vi "simulation.vi"(1 "Stop signaller":refnum<class "Signaller.lvclass">, 2 "Simulation config action queue":refnum<queue>, 3 "Frequency refnum":refnum<vi>, 4 "Data input file refnum":refnum<vi>) -> ()   [LabVIEW 2019]
uses:
  Fit Parameters.ctl
  Physical Constants.ctl
  Internal Parameters.ctl
  System parameters.ctl
  Motor controller/Signaller/Signaller.lvclass
  <vilib>/Platform/TimedLoop/XDataNode/timing_clust.ctl
  <vilib>/Platform/TimedLoop/XDataNode/nitl_modes.ctl
  <vilib>/Platform/TimedLoop/XDataNode/wakeup.ctl
  <vilib>/Platform/TimedLoop/scheduler/LVUserAPI/_suppVIs/Create_1kHz_TSource.vi
  <vilib>/Utility/file.llb/Write Delimited Spreadsheet (string).vi
  <vilib>/Utility/config.llb/Read Key (Path).vi
  <vilib>/Utility/config.llb/Read Key (Boolean).vi
  <vilib>/Utility/config.llb/Read Key (Double).vi
  <vilib>/Utility/config.llb/Read Key (U32).vi
  <vilib>/Utility/config.llb/Read Key (I32).vi
  <vilib>/Utility/config.llb/Write Key (Path).vi
  <vilib>/Utility/config.llb/Write Key (Boolean).vi
  <vilib>/Utility/config.llb/Write Key (Double).vi
  <vilib>/Utility/config.llb/Write Key (U32).vi
  <vilib>/Utility/config.llb/Write Key (I32).vi
  <vilib>/platform/TimedLoop/XDataNode/XDataNode.xnode
  <vilib>/Platform/TimedLoop/XDataNode/XDNodeRunTimeDep.lvlib
  <vilib>/Utility/config.llb/NI_LVConfig.lvlib
panel:
  in  "Precision":i32=100 min=1
  in  "Sweep error":dbl=0.01 min=0.0 format="%#_13g"
  out "Start time":timestamp
  out "Polarization (unfuzzed)":dbl
  in  "Thermal fluctuations":dbl=0.01 min=0.0
  out "Pn (noisy)":dbl
  in  "System parameters":T1={"Frequency (GHz)"=140.2, "System temperature (K)"=1.0, "Beam current (nA)"=100.0}
  out "Internal parameters":T2={"Pe"=-1.0, "Pn"=0.0, "Alpha"=0.0, "Beta"=0.0, "C"=0.000136073, "Phi"=0.0, "Pe0"=-1.0, "Dose"=0.0, "Temperature"=1.0}
  in  "Physical constants":T3={"T1e (s)"=0.03, "T1n (s)"=1500.0}
  in  "Fit parameters":T4={"A"=0.572086, "S"=0.0835606, "M1"=140.286, "M2"=140.486}
  in  "Launch fit parameters chooser":bool
  out "Elapsed time (s)":dbl
  in  "Reset simulation":bool
  in  "Paused":bool=TRUE
  out "Current time (simulated)":timestamp format="%<%H:%M:%S\n%B %d, %Y>T"
  in  "Stop simulation":bool
  in  "Data output file":path
  out "Polarization":dbl
  in  "Beam on":bool
  in  "Time per second (s)":dbl=1.0
  out "Seconds until next data":u32
  in  "# Sweeps":u32=250
  in  "Add 30 minutes":bool
  in  "30 minutes":bool
  in  "15 minutes":bool
  in  "5 minutes":bool
  in  "Time scale (min)":i64=5 min=1
  out "Polarization vs time":cluster{timestamp[], dbl[]}(graph)
  # "Advanced data and controls"
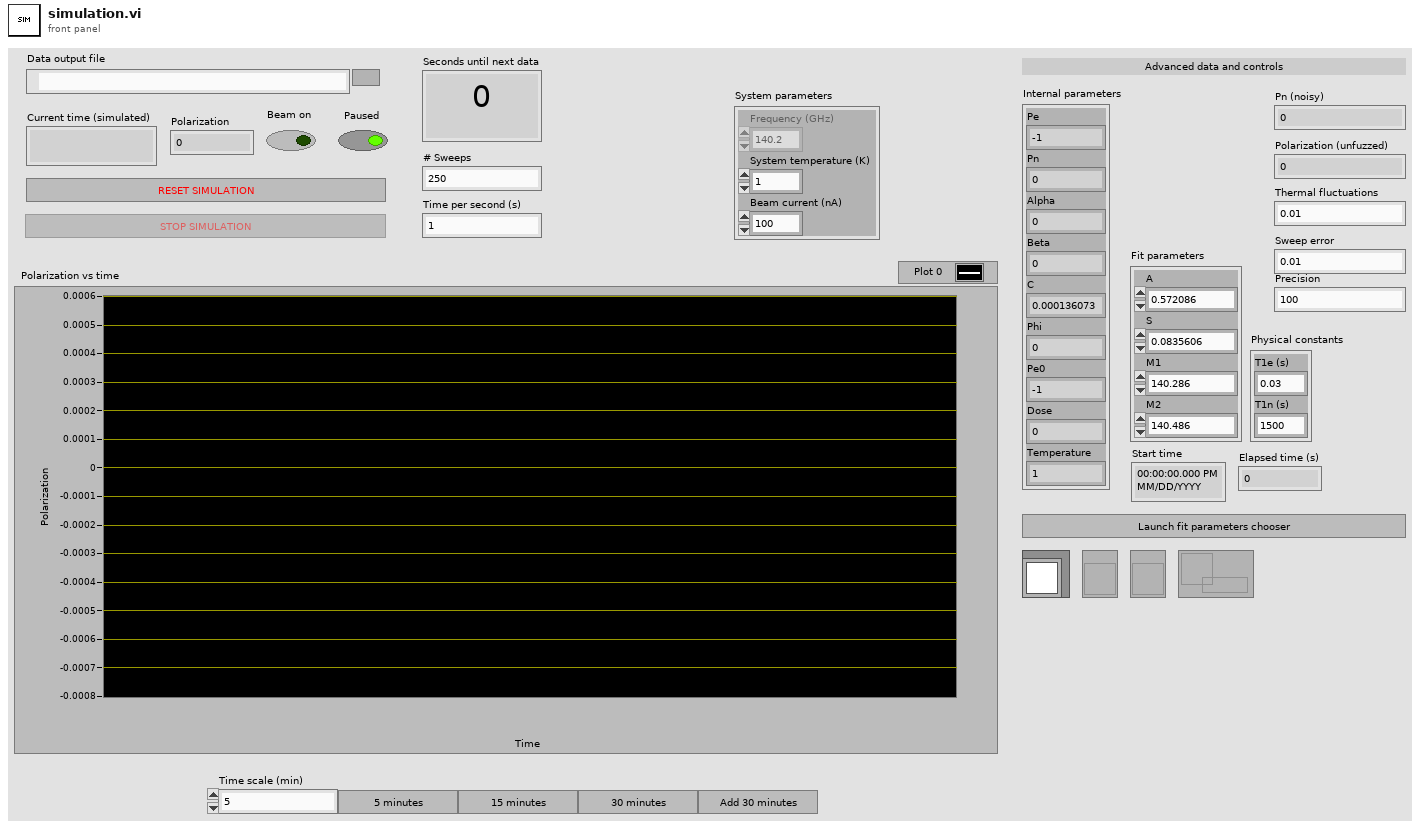
[diagram p1: front panel]
types:
  T1 = typedef "System parameters.ctl" = cluster{"Frequency (GHz)":dbl, "System temperature (K)":dbl, "Beam current (nA)":dbl}
  T2 = typedef "Internal Parameters.ctl" = cluster{"Pe":dbl, "Pn":dbl, "Alpha":dbl, "Beta":dbl, "C":dbl, "Phi":dbl, "Pe0":dbl, "Dose":dbl, "Temperature":dbl}
  T3 = typedef "Physical Constants.ctl" = cluster{"T1e (s)":dbl, "T1n (s)":dbl}
  T4 = typedef "Fit Parameters.ctl" = cluster{"A":dbl, "S":dbl, "M1":dbl, "M2":dbl}
  T5 = enum8{"Enabled", "Disabled", "Disabled and Grayed Out"}
  T6 = typedef "Semaphore RefNum" = refnum<k1>
  T7 = typedef "XDNodeRunTimeDep.lvlib/timing_clust.ctl" = cluster{"Expected End [f-1]":u64, "Actual End [f-1]":u64, "Finished Late? [f-1]":bool, "Expected End [i-1]":u64, "Actual End [i-1]":u64, "Finished Late? [i-1]":bool, "Expected Start [i]":u64, "Actual Start [i]":u64, "Expected Start [f]":u64, "Actual Start [f]":u64, "Source Name":string, "Structure Name":string, "Period":i64, "Deadline":i64, "Offset":i64, "Start":i64, "Priority":i32, "Timeout":i32, "Mode":T8, "Wakeup Reason":T9, "Error":errorcluster, "Source Type":string, "Secondary Source Type":string, "Global End Time":u64, "Global Start Time":u64, "Frame Duration":u64, "Iteration Duration":u64, "Assigned CPU":i32, "I/O Scan Engine Mode":u32}
  T8 = typedef "XDNodeRunTimeDep.lvlib/nitl_modes.ctl" = enum32{"No Change", "Process missed periods, maintain original phase", "Discard missed periods, maintain original phase", "Process missed periods, ignore original phase", "Discard missed periods, ignore original phase"}
  T9 = typedef "XDNodeRunTimeDep.lvlib/wakeup.ctl" = enum32{"Normal", "Aborted", "Asynchronous wakeup", "Timing source error", "Timed loop error", "Timeout"}
  T10 = typedef "LVRangeTypeDef.ctl" = cluster{"Minimum":dbl, "Maximum":dbl, "Increment":dbl, "Minor Increment":dbl, "Start":dbl}
  T11 = typedef "NI_LVConfig.lvlib/Config Data RefNum.ctl" = refnum<k1>
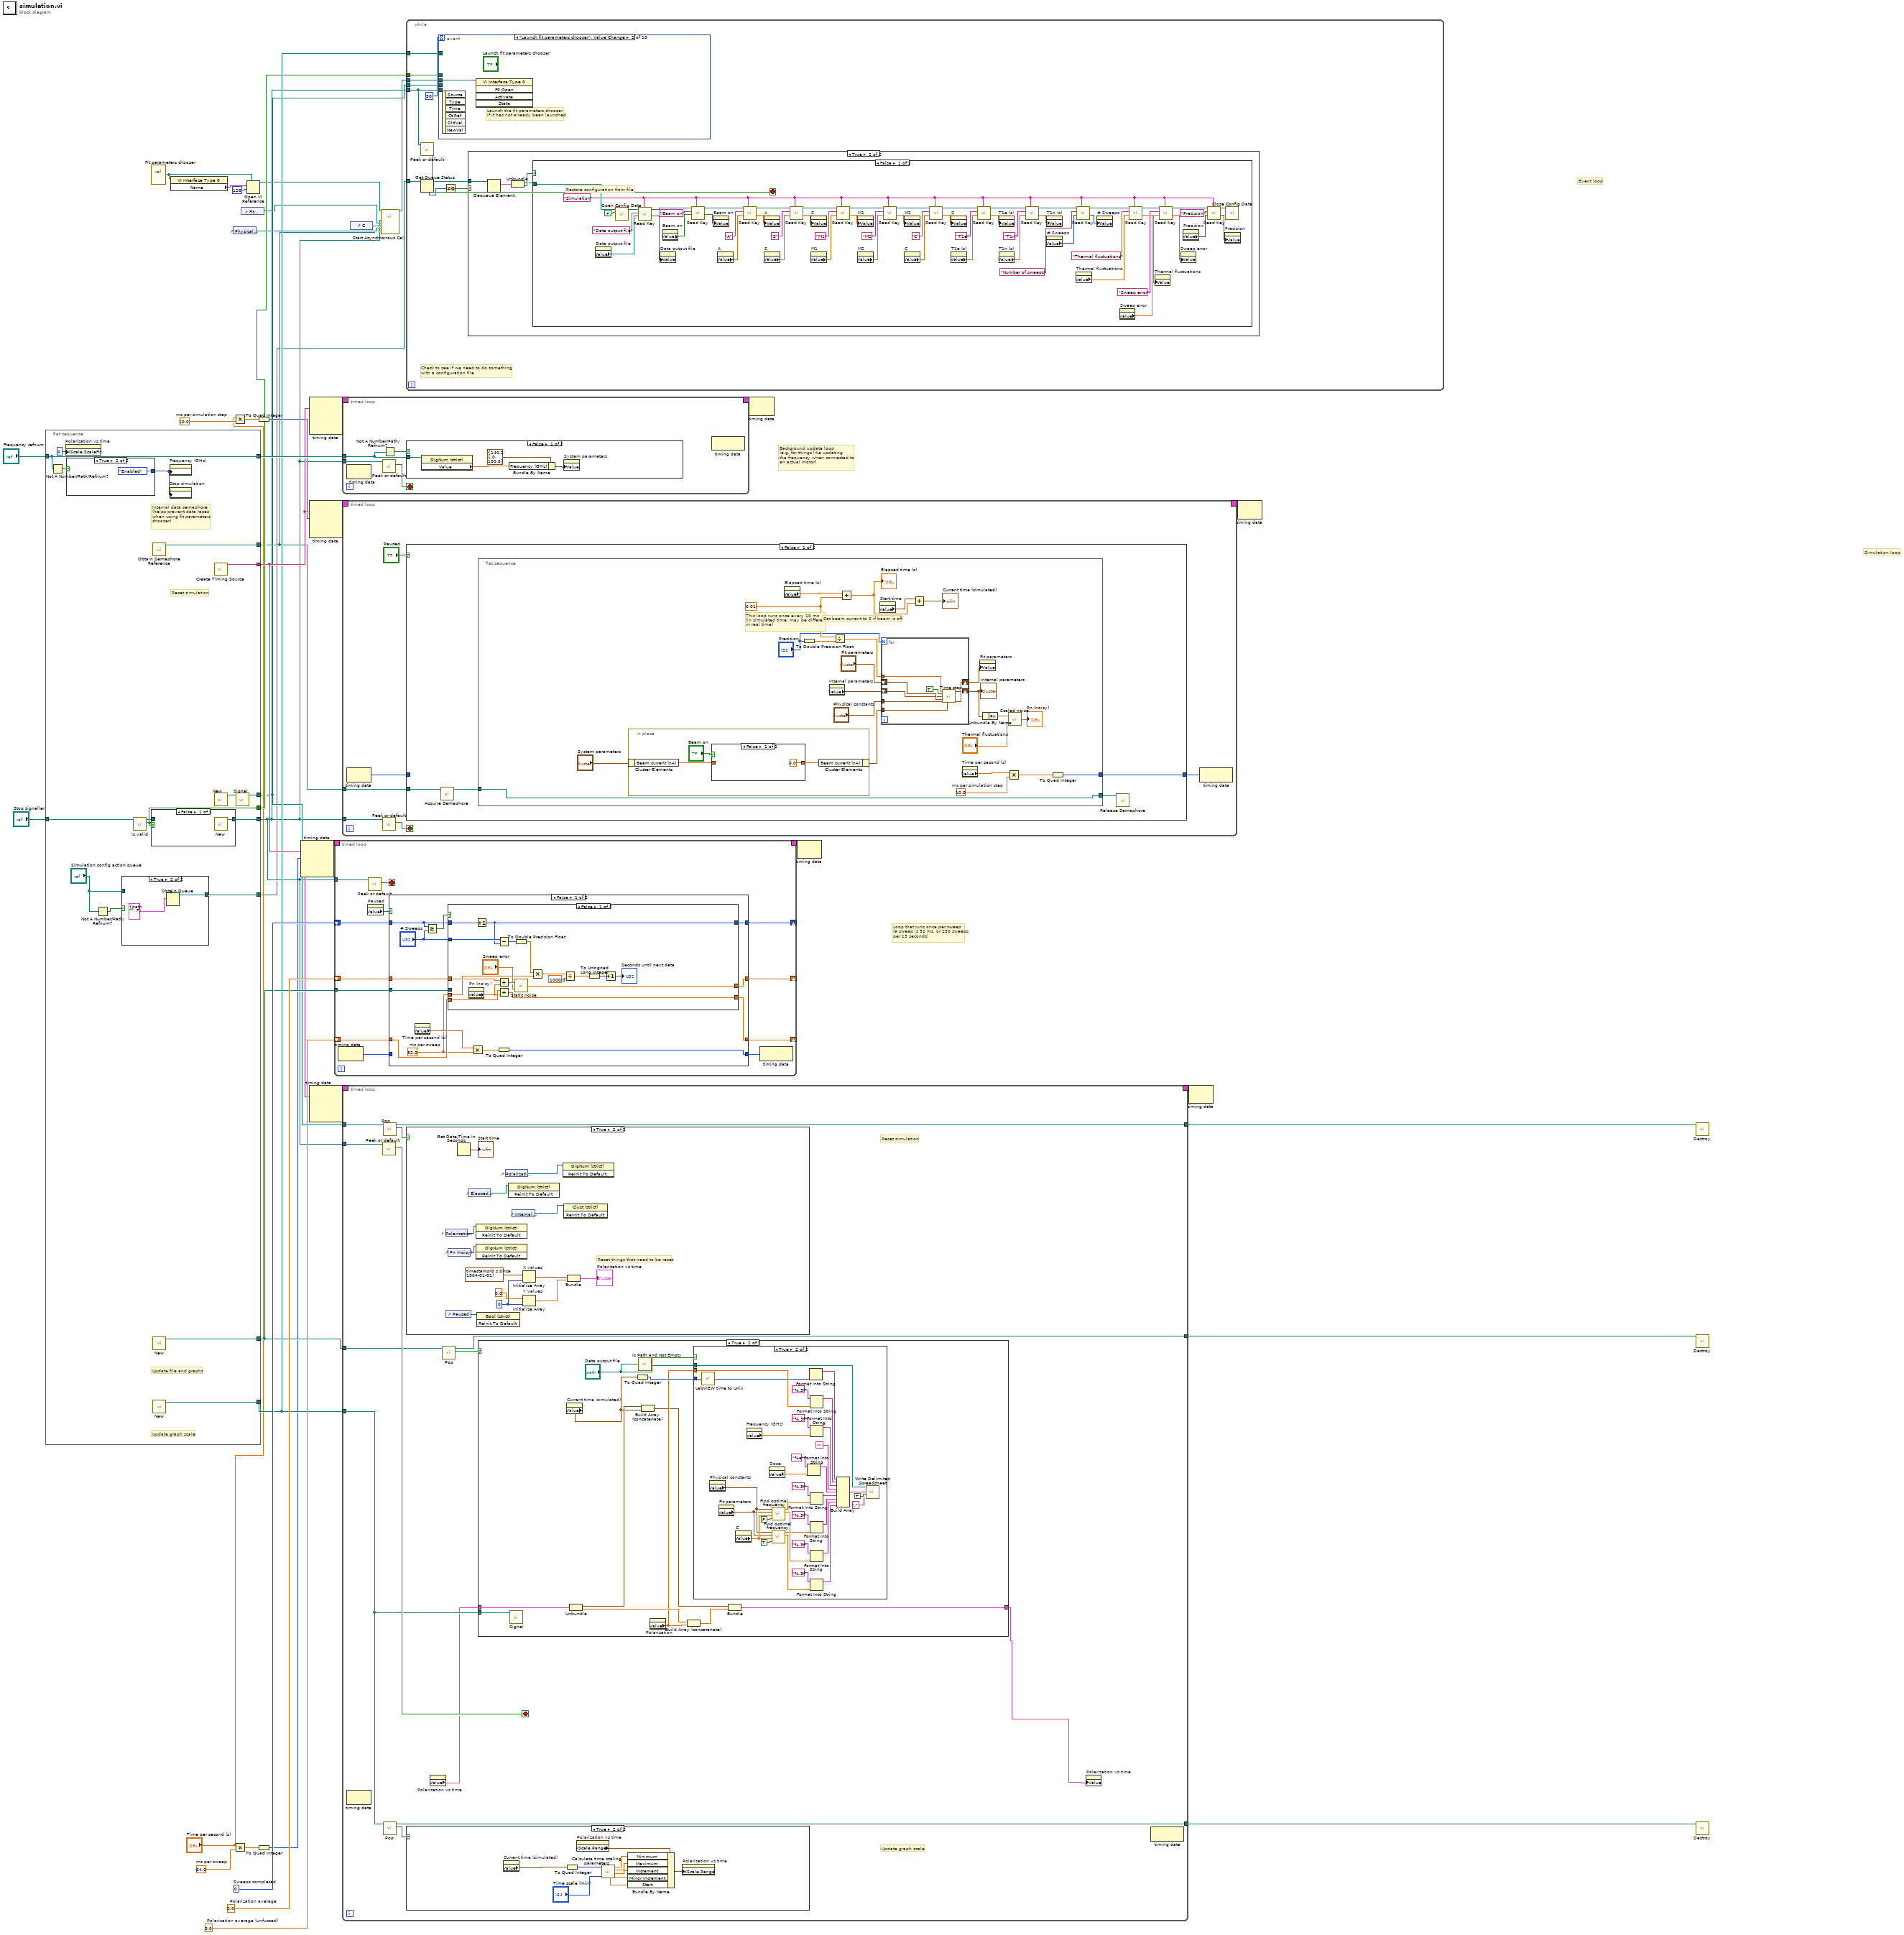
[diagram p0: block diagram]
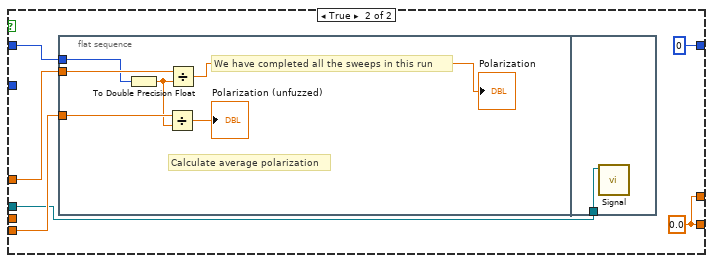
[diagram p6: hidden frame]
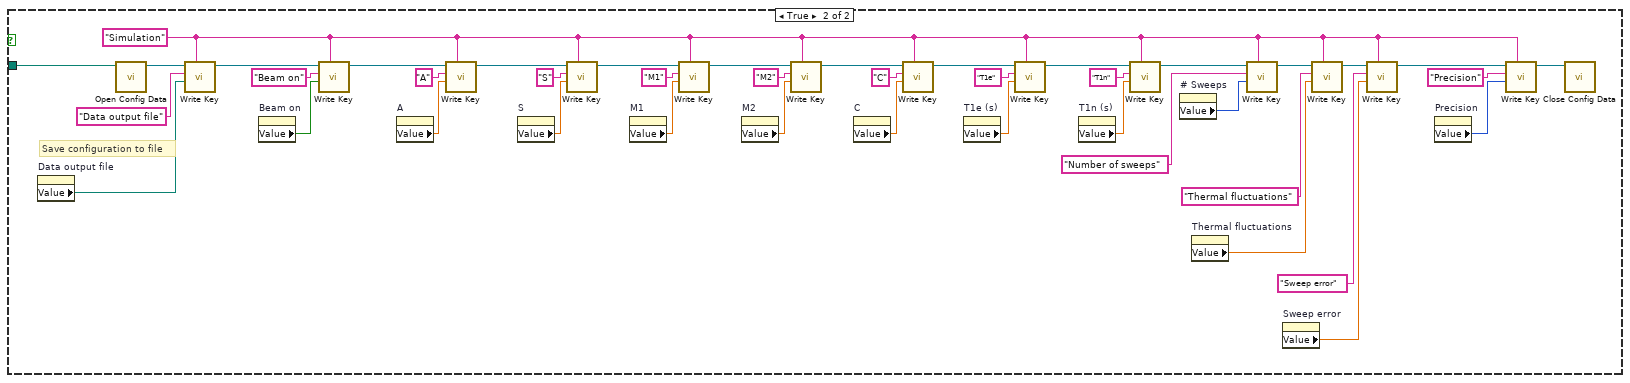
[diagram p12: hidden frame]
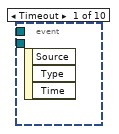
[diagram p13: hidden frame]
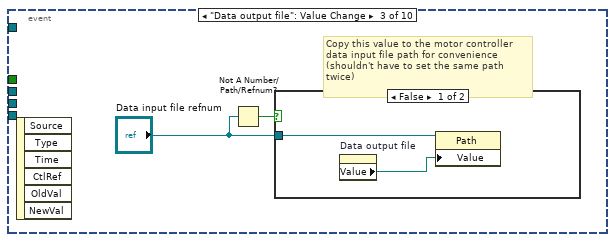
[diagram p14: hidden frame]
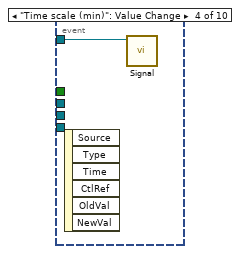
[diagram p16: hidden frame]
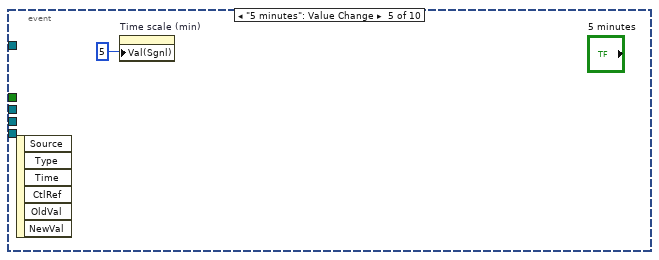
[diagram p17: hidden frame]
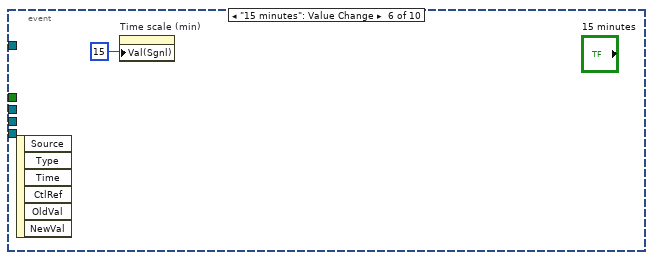
[diagram p18: hidden frame]
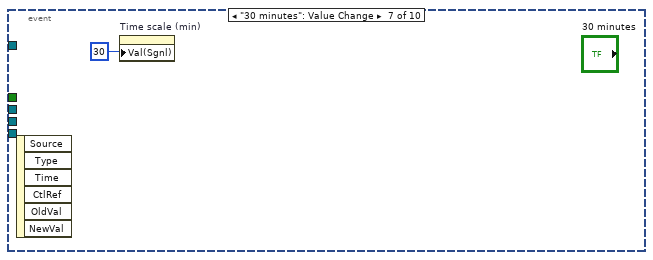
[diagram p19: hidden frame]
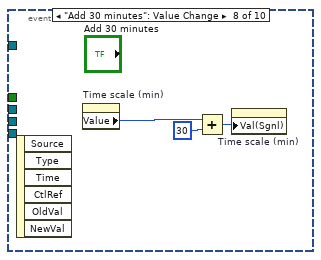
[diagram p20: hidden frame]
diagram:
  w16 = 64.0  # ms per sweep
  w20 = 10.0  # ms per simulation step
  w30 = 0.0  # Polarization average (unfuzzed)
  w31 = 0.0  # Polarization average
  w32 = u32 0  # Sweeps completed
  # "Loop that runs once per sweep\n(a sweep is 52 ms, or 250 sweeps\nper 13 seconds)"
  # "Background update loop\n(e.g. for things like updating\nthe frequency when connected to\nan actual motor)"
  # "Event loop"
  # "Simulation loop"
  n1 = flat-sequence {
    tunnel: "Frequency refnum" -> [w56]
    tunnel: [w48] -> w3
    tunnel: [w56] -> w39
    tunnel: [w53] -> w28
    tunnel: [w52] -> w22
    tunnel: "Stop signaller" -> [w50]
    tunnel: [w51] -> w23
    tunnel: [w47] -> w21
    tunnel: [w45] -> w12
    tunnel: [w44] -> w4
    tunnel: [w42] -> w1
    frame #0 {
      # "Internal data semaphore\n(helps prevent data races\nwhen using fit parameters\nchooser)"
      # "Reset simulation"
      # "Update graph scale"
      # "Update file and graphs"
      n2 = Not A Number/Path/Refnum?(number/path/refnum=w56) -> (NaN/Path/Refnum?=w57:bool)
      n3 = property on="Polarization vs time" class="XYGraph (strict)"("XScale.ScaleFit"=u8 0 ("X Scale.Scale Fit")) -> ()  [unwired: 2 in, 2 out]
      n4 = case shown="True" w57 {
        tunnel: [T5."Disabled and Grayed Out" ("Disabled") T5."Enabled" ("Disabled")] -> w54
        frame False {
        }
        frame True {
        }
      }
      n5 = Not A Number/Path/Refnum?(number/path/refnum="Simulation config action queue") -> (NaN/Path/Refnum?=w43:bool)
      n6 = case shown="True" w43 {
        tunnel: [w58 w59] -> w42
        tunnel: "Simulation config action queue" -> [w58 _]
        frame False {
        }
        frame True {
          n7 = Obtain Queue(element data type=cluster{path, bool} {path "", FALSE}) -> (queue out=w59:refnum<queue>)  [unwired: 4 in, 2 out]
        }
      }
      n8 = call "Is valid.vi"("Signaller in"=w50) -> ("Is valid?"=w47:bool, "Signaller out"=w49:refnum<class "Signaller.lvclass">)  [unwired: 8 in, 1 out]
      n9 = case shown="False" w47 {
        tunnel: w49 -> [_ w62]
        tunnel: [w61 w62] -> w48
        frame False {
          n10 = call "New.vi"() -> ("Signaller out"=w61:refnum<class "Signaller.lvclass">)  [unwired: 11 in]
        }
        frame True {
        }
      }
      n11 = call <vilib>:"Obtain Semaphore Reference.vi"() -> ("semaphore"=w44:T6)  [unwired: 5 in, 2 out]
      n12 = call "New.vi"() -> ("Signaller out"=w53:refnum<class "Signaller.lvclass">)  [unwired: 11 in]
      n13 = call "New.vi"() -> ("Signaller out"=w52:refnum<class "Signaller.lvclass">)  [unwired: 11 in]
      n14 = property on="Frequency (GHz)" class="DigNum (strict)"("DisabledEnum"=w54) -> ()  [unwired: 2 in, 2 out]
      n15 = property on="Stop simulation" class="Bool"("DisabledEnum"=w54) -> ()  [unwired: 2 in, 2 out]
      n16 = call-poly <vilib>:"Create Timing Source.vi"() -> ("name (out)"=w51:string)  [unwired: 10 in, 1 out]
      n17 = call "New.vi"() -> ("Signaller out"=w46:refnum<class "Signaller.lvclass">)  [unwired: 11 in]
      n18 = call "Signal.vi"("Signaller in"=w46) -> ("Signaller out"=w45:refnum<class "Signaller.lvclass">)  [unwired: 9 in, 1 out]
    }
  }
  n19 = vi-ref "Fit parameters chooser.vi"() -> (w7:refnum<vi>)
  n20 = property class="VI Interface Type 0"(reference=w7) -> ("Name"=w8:string)  [unwired: 1 in, 2 out]
  n21 = control-ref of="Physical constants"() -> (w11:refnum<vi>)
  n22 = Multiply(x="Time per second (s)", y=w20) -> (x*y=w19:dbl)
  n23 = Multiply(x="Time per second (s)", y=w16) -> (x*y=w15:dbl)
  n24 = control-ref of="Fit parameters"() -> (w9:refnum<vi>)
  n25 = Open VI Reference(type specifier VI Refnum (for type only)=w7, vi path=w8, options=128) -> (vi reference=w5:refnum<vi>)  [unwired: 3 in, 1 out]
  n26 = To Quad Integer(1:w19) -> (0:w18:i64)
  n27 = To Quad Integer(1:w15) -> (0:w14:i64)
  n28 = node-c288(w23, w14) -> (w34:T7)  [unwired: 2 in]
  n29 = node-c288(w23) -> (w36:T7)  [unwired: 3 in]
  n30 = node-c288(w23, w18) -> (w38:T7)  [unwired: 2 in]
  n31 = node-c288(w23) -> (w27:T7)  [unwired: 3 in]
  n32 = timed-loop {
    timing: w34 -> [_]
    timing-out: [_] -> w33
    tunnel: w3 -> [w75]
    shift-right: [w73] -> _
    shift-left: w32 -> [w74]
    shift-right: [w71] -> _
    shift-left: w31 -> [w72]
    shift-right: [w69] -> _
    shift-left: w30 -> [w70]
    tunnel: w28 -> [w68]
    stop <- w76 stop-if-true
    n33 = node-c288() -> (w65:i64)  [unwired: 1 in]
    n34 = property on="Paused" class="Bool (strict)"() -> ("Value"=w66:bool)  [unwired: 2 in, 2 out]
    n35 = call "Peek or default.vi"("Signaller in"=w75) -> ("Has signal?"=w76:bool)  [unwired: 8 in, 2 out]
    n36 = case shown="False" w66 {
      tunnel: w74 -> [w88 w124]
      tunnel: [w87 w124] -> w73
      tunnel: w72 -> [w85 w123]
      tunnel: [w84 w123] -> w71
      tunnel: w70 -> [w83 w122]
      tunnel: [w82 w122] -> w69
      tunnel: w68 -> [w81 _]
      tunnel: [w79 w121] -> w67
      tunnel: w65 -> [_ w121]
      frame False {
        w77 = 52.0  # ms per sweep
        n37 = property on="Time per second (s)" class="DigNum (strict)"() -> ("Value"=w80:dbl)  [unwired: 2 in, 2 out]
        n38 = Greater Or Equal?(x=w88, y="# Sweeps") -> (x >= y?=w89:bool)
        n39 = case shown="False" w89 {
          tunnel: w88 -> [w106 w111]
          tunnel: [w105 u32 0] -> w87
          tunnel: "# Sweeps" -> [w107 _]
          tunnel: w85 -> [w103 w112]
          tunnel: [w101 w109] -> w84
          tunnel: w83 -> [w99 w110]
          tunnel: [w97 w109] -> w82
          tunnel: w81 -> [_ w108]
          tunnel: w77 -> [w95 _]
          frame False {
            n40 = property on="Pn (noisy)" class="DigNum (strict)"() -> ("Value"=w98:dbl)  [unwired: 2 in, 2 out]
            n41 = Increment(x=w106) -> (x+1=w105:u32)
            n42 = Subtract(x=w107, y=w105) -> (x-y=w96:u32)
            n43 = Add(x=w103, y=w98) -> (x+y=w102:dbl)
            n44 = Add(x=w99, y=w98) -> (x+y=w97:dbl)
            n45 = To Double Precision Float(number=w96) -> (double precision float=w94:dbl)
            n46 = call "Static noise.vi"("Fraction"="Sweep error", "Input"=w102) -> ("Output with noise"=w101:dbl)
            n47 = Multiply(x=w94, y=w95) -> (x*y=w93:dbl)
            n48 = Divide(x=w93, y=1000.0) -> (x/y=w91:dbl)
            n49 = To Unsigned Long Integer(number=w91) -> (unsigned 32bit integer=w90:u32)
            n50 = Increment(x=w90) -> (x+1=→"Seconds until next data":u32)
          }
          frame True {
            w109 = 0.0
            n51 = flat-sequence {
              tunnel: w112 -> [w119]
              tunnel: w111 -> [w118]
              tunnel: w110 -> [w116]
              tunnel: w108 -> [w120]
              frame #0 {
                # "Calculate average polarization"
                # "We have completed all the sweeps in this run"
                n52 = To Double Precision Float(number=w118) -> (double precision float=w115:dbl)
                n53 = Divide(x=w116, y=w115) -> (x/y=→"Polarization (unfuzzed)":dbl)
                n54 = Divide(x=w119, y=w115) -> (x/y=→"Polarization":dbl)
              }
              frame #1 {
                n55 = call "Signal.vi"("Signaller in"=w120) -> ()  [unwired: 9 in, 2 out]
              }
            }
          }
        }
        n56 = Multiply(x=w80, y=w77) -> (x*y=w78:dbl)
        n57 = To Quad Integer(1:w78) -> (0:w79:i64)
      }
      frame True {
      }
    }
    n58 = node-c288(w67) -> ()  [unwired: 1 out]
  }
  n59 = timed-loop {
    tunnel: w39 -> [w132]
    tunnel: w3 -> [w130]
    timing: w36 -> [_]
    timing-out: [_] -> w35
    stop <- w131 stop-if-true
    n60 = node-c288() -> ()  [unwired: 1 in, 1 out]
    n61 = call "Peek or default.vi"("Signaller in"=w130) -> ("Has signal?"=w131:bool)  [unwired: 8 in, 2 out]
    n62 = Not A Number/Path/Refnum?(number/path/refnum=w132) -> (NaN/Path/Refnum?=w133:bool)
    n63 = case shown="False" w133 {
      tunnel: w132 -> [w139 _]
      frame False {
        n64 = property class="DigNum (strict)"(reference=w139) -> ("Value"=w136:dbl)  [unwired: 1 in, 2 out]
        n65 = Bundle By Name(cluster=T1 {"Frequency (GHz)"=140.2, "System temperature (K)"=1.0, "Beam current (nA)"=100.0} ("System parameters"), "Frequency (GHz)"=w136) -> (w138:T1)
        n66 = property on="System parameters" class="Clust (strict)"("Value"=w138) -> ()  [unwired: 2 in, 2 out]
      }
      frame True {
      }
    }
    n67 = node-c288() -> ()  [unwired: 1 in, 1 out]
  }
  n68 = timed-loop {
    tunnel: w3 -> [w144]
    timing: w38 -> [_]
    timing-out: [_] -> w37
    tunnel: w4 -> [w140]
    stop <- w145 stop-if-true
    n69 = node-c288() -> (w141:i64)  [unwired: 1 in]
    n70 = call "Peek or default.vi"("Signaller in"=w144) -> ("Has signal?"=w145:bool)  [unwired: 8 in, 2 out]
    n71 = case shown="False" "Paused" {
      tunnel: [w149 w186] -> w143
      tunnel: w141 -> [_ w186]
      tunnel: w140 -> [w148 _]
      frame False {
        n72 = call <vilib>:"Acquire Semaphore.vi"("semaphore"=w148) -> ("semaphore out"=w147:T6)  [unwired: 4 in, 2 out]
        n73 = flat-sequence {
          tunnel: [w158] -> w149
          tunnel: w147 -> [w156]
          tunnel: [w156] -> w146
          frame #0 {
            w160 = 10.0  # ms per simulation step
            w153 = 0.01
            # "This loop runs once every 10 ms\n(in simulated time; may be different\nin real time)"
            # "Set beam current to 0 if beam is off"
            n74 = in-place {
              n75 = in-place-cluster #1("System parameters") -> ("Beam current (nA)"=w182:dbl)
              n76 = case shown="False" "Beam on" {
                tunnel: w182 -> [_ w185]
                tunnel: [0.0 ("Beam current (nA)") w185] -> w181
                frame False {
                }
                frame True {
                }
              }
              n77 = in-place-cluster #1("Beam current (nA)"=w181) -> (w165:T1)
            }
            n78 = property on="Elapsed time (s)" class="DigNum (strict)"() -> ("Value"=w172:dbl)  [unwired: 2 in, 2 out]
            n79 = To Double Precision Float(number="Precision") -> (double precision float=w152:dbl)
            n80 = property on="Internal parameters" class="Clust (strict)"() -> ("Value"=w154:T2)  [unwired: 2 in, 2 out]
            n81 = Divide(x=w153, y=w152) -> (x/y=w150:dbl)
            n82 = Add(x=w172, y=w153) -> (x+y=w162:dbl)
            "Elapsed time (s)" <- w162
            n83 = property on="Start time" class="AbsTime (strict)"() -> ("Value"=w163:timestamp)  [unwired: 2 in, 2 out]
            n84 = for {
              N: "Precision" -> [_]
              tunnel: "Physical constants" -> [w180]
              tunnel: w165 -> [w178]
              tunnel: w150 -> [w176]
              shift-right: [w175] -> w157
              shift-left: "Fit parameters" -> [w179]
              shift-right: [w174] -> w155
              shift-left: w154 -> [w173]
              n85 = call "Time step.vi"("Time (s)"=w176, "Microwave on"=TRUE, "Internal parameters in"=w173, "Fit parameters"=w179, "Physical constants"=w180, "System parameters"=w178) -> ("Internal parameters out"=w174:T2, "Fit parameters out"=w175:T4)  [unwired: 8 in]
            }
            "Internal parameters" <- w155
            n86 = Add(x=w163, y=w162) -> (x+y=→"Current time (simulated)":timestamp)
            n87 = property on="Time per second (s)" class="DigNum (strict)"() -> ("Value"=w159:dbl)  [unwired: 2 in, 2 out]
            n88 = property on="Fit parameters" class="Clust (strict)"("Value"=w157) -> ()  [unwired: 2 in, 2 out]
            n89 = Unbundle By Name(w155) -> ("Pn"=w170:dbl)
            n90 = Multiply(x=w159, y=w160) -> (x*y=w161:dbl)
            n91 = call "Scaled noise.vi"("Fraction"="Thermal fluctuations", "Input"=w170) -> ("Output with noise"=→"Pn (noisy)":dbl)
            n92 = To Quad Integer(1:w161) -> (0:w158:i64)
          }
        }
        n93 = call <vilib>:"Release Semaphore.vi"("semaphore"=w146) -> ()  [unwired: 5 in, 2 out]
      }
      frame True {
      }
    }
    n94 = node-c288(w143) -> ()  [unwired: 1 out]
  }
  n95 = timed-loop {
    tunnel: w3 -> [w202]
    tunnel: w28 -> [w201]
    tunnel: [w200] -> w29
    timing: w27 -> [_]
    timing-out: [_] -> w26
    tunnel: w22 -> [w197]
    tunnel: [w198] -> w25
    tunnel: w12 -> [w196]
    tunnel: [w194] -> w13
    stop <- w203 stop-if-true
    # "Update graph scale"
    # "Reset simulation"
    n96 = node-c288() -> ()  [unwired: 1 in, 1 out]
    n97 = call "Peek or default.vi"("Signaller in"=w202) -> ("Has signal?"=w203:bool)  [unwired: 8 in, 2 out]
    n98 = call "Pop.vi"("Signaller in"=w196) -> ("Has signal"=w195:bool, "Signaller out"=w194:refnum<class "Signaller.lvclass">)  [unwired: 8 in, 1 out]
    n99 = call "Pop.vi"("Signaller in"=w197) -> ("Has signal"=w199:bool, "Signaller out"=w198:refnum<class "Signaller.lvclass">)  [unwired: 8 in, 1 out]
    n100 = case shown="True" w195 {
      frame False {
      }
      frame True {
        w208 = 0 ("dimension size")
        # "Reset things that need to be reset"
        n101 = control-ref of="Polarization"() -> (w215:refnum<vi>)
        n102 = control-ref of="Paused"() -> (w205:refnum<vi>)
        n103 = control-ref of="Pn (noisy)"() -> (w214:refnum<vi>)
        n104 = Get Date/Time In Seconds() -> (seconds since 1Jan1904=→"Start time":timestamp)
        n105 = control-ref of="Elapsed time (s)"() -> (w213:refnum<vi>)
        n106 = invoke class="DigNum (strict)" method="Reinit To Default"(reference=w215) -> ()  [unwired: 2 in, 3 out]
        n107 = invoke class="DigNum (strict)" method="Reinit To Default"(reference=w214) -> ()  [unwired: 2 in, 3 out]
        n108 = invoke class="Bool (strict)" method="Reinit To Default"(reference=w205) -> ()  [unwired: 2 in, 3 out]
        n109 = control-ref of="Polarization (unfuzzed)"() -> (w216:refnum<vi>)
        n110 = invoke class="DigNum (strict)" method="Reinit To Default"(reference=w213) -> ()  [unwired: 2 in, 3 out]
        n111 = control-ref of="Internal parameters"() -> (w212:refnum<vi>)
        n112 = Initialize Array "X values"(timestamp(0 s since 1904-01-01), w208) -> (w209:timestamp[])
        n113 = Initialize Array "Y values"(0.0, w208) -> (w210:dbl[])
        n114 = invoke class="DigNum (strict)" method="Reinit To Default"(reference=w216) -> ()  [unwired: 2 in, 3 out]
        n115 = invoke class="Clust (strict)" method="Reinit To Default"(reference=w212) -> ()  [unwired: 2 in, 3 out]
        n116 = Bundle(w209, w210) -> (→"Polarization vs time":cluster{timestamp[], dbl[]})  [unwired: 1 in]
      }
    }
    n117 = case shown="True" w199 {
      frame False {
      }
      frame True {
        n118 = property on="Current time (simulated)" class="AbsTime (strict)"() -> ("Value"=w218:timestamp)  [unwired: 2 in, 2 out]
        n119 = To Quad Integer(1:w218) -> (0:w220:i64)
        n120 = property on="Polarization vs time" class="XYGraph (strict)"() -> ("XScale.Range"=w221:T10)  [unwired: 2 in, 2 out]
        n121 = call "Calculate time scaling parameters.vi"("Time"=w220, "Time scale (minutes)"="Time scale (min)") -> ("Minimum"=w224:dbl, "Maximum"=w225:dbl, "Increment"=w226:dbl, "Minor increment"=w227:dbl, "Start"=w223:dbl)  [unwired: 1 in]
        n122 = Bundle By Name(cluster=w221, "Minimum"=w224, "Maximum"=w225, "Increment"=w226, "Minor Increment"=w227, "Start"=w223) -> (w222:T10)
        n123 = property on="Polarization vs time" class="XYGraph (strict)"("XScale.Range"=w222) -> ()  [unwired: 2 in, 2 out]
      }
    }
    n124 = property on="Polarization vs time" class="XYGraph (strict)"() -> ("Value"=w192:cluster{timestamp[], dbl[]})  [unwired: 2 in, 2 out]
    n125 = call "Pop.vi"("Signaller in"=w201) -> ("Has signal"=w204:bool, "Signaller out"=w200:refnum<class "Signaller.lvclass">)  [unwired: 8 in, 1 out]
    n126 = case shown="True" w204 {
      tunnel: w192 -> [w230 w240]
      tunnel: [w230 w233] -> w193
      tunnel: w197 -> [_ w231]
      frame False {
      }
      frame True {
        n127 = call "Signal.vi"("Signaller in"=w231) -> ()  [unwired: 9 in, 2 out]
        n128 = property on="Current time (simulated)" class="AbsTime (strict)"() -> ("Value"=w232:timestamp)  [unwired: 2 in, 2 out]
        n129 = Unbundle(w240) -> (w239:timestamp[], w238:dbl[])
        n130 = To Quad Integer(1:w232) -> (0:w237:i64)
        n131 = call <vilib>:"Is Path and Not Empty.vi"("path"="Data output file") -> ("Is Path and Not Empty?"=w242:bool)  [unwired: 4 in]
        n132 = Build Array (concatenate)(w239, w232) -> (w234:timestamp[])
        n133 = property on="Polarization" class="DigNum (strict)"() -> ("Value"=w236:dbl)  [unwired: 2 in, 2 out]
        n134 = Build Array (concatenate)(w238, w236) -> (w235:dbl[])
        n135 = case shown="True" w242 {
          tunnel: "Data output file" -> [_ w273]
          tunnel: w237 -> [_ w272]
          tunnel: w236 -> [_ w269]
          frame False {
          }
          frame True {
            n136 = call "LabVIEW time to Unix.vi"("LabVIEW time"=w272) -> ("Unix time"=w271:i64)
            n137 = property on="Physical constants" class="Clust (strict)"() -> ("Value"=w250:T3)  [unwired: 2 in, 2 out]
            n138 = property on="Fit parameters" class="Clust (strict)"() -> ("Value"=w249:T4)  [unwired: 2 in, 2 out]
            n139 = property on="C" class="DigNum (strict)"() -> ("Value"=w251:dbl)  [unwired: 2 in, 2 out]
            n140 = property on="Frequency (GHz)" class="DigNum (strict)"() -> ("Value"=w261:dbl)  [unwired: 2 in, 2 out]
            n141 = property on="Dose" class="DigNum (strict)"() -> ("Value"=w265:dbl)  [unwired: 2 in, 2 out]
            n142 = call "Find optimal frequency.vi"("Find optimal for negative polarization?"=FALSE, "C"=w251, "Fit parameters"=w249, "Physical constants"=w250) -> ("Steady state at optimal frequency"=w246:dbl, "Optimal frequency (GHz)"=w256:dbl)  [unwired: 6 in]
            n143 = call "Find optimal frequency.vi"("Find optimal for negative polarization?"=TRUE, "C"=w251, "Fit parameters"=w249, "Physical constants"=w250) -> ("Steady state at optimal frequency"=w244:dbl, "Optimal frequency (GHz)"=w253:dbl)  [unwired: 6 in]
            n144 = Format Into String(format string="%e", w265) -> (resulting string=w263:string)  [unwired: 2 in, 1 out]
            n145 = Format Into String(w271) -> (resulting string=w270:string)  [unwired: 3 in, 1 out]
            n146 = Format Into String(format string="%.3f", w269) -> (resulting string=w267:string)  [unwired: 2 in, 1 out]
            n147 = Format Into String(format string="%.3f", w261) -> (resulting string=w260:string)  [unwired: 2 in, 1 out]
            n148 = Format Into String(format string="%.3f", w256) -> (resulting string=w255:string)  [unwired: 2 in, 1 out]
            n149 = Format Into String(format string="%.3f", w253) -> (resulting string=w252:string)  [unwired: 2 in, 1 out]
            n150 = Format Into String(format string="%.3f", w246) -> (resulting string=w245:string)  [unwired: 2 in, 1 out]
            n151 = Format Into String(format string="%.3f", w244) -> (resulting string=w243:string)  [unwired: 2 in, 1 out]
            n152 = Build Array(w270, w267, w260, "", w263, w255, w252, w245, w243) -> (w274:string[])
            n153 = call-poly <vilib>:"Write Delimited Spreadsheet.vi"("file path (dialog if empty)"=w273, "1D data"=w274, "append to file? (new file:F)"=TRUE ("append to file? (F)"), "delimiter (\\t)"="," ("delimiter (\\t)")) -> ()  [unwired: 10 in, 2 out]
          }
        }
        n154 = Bundle(w234, w235) -> (w233:cluster{timestamp[], dbl[]})  [unwired: 1 in]
      }
    }
    n155 = property on="Polarization vs time" class="XYGraph (strict)"("Value"=w193) -> ()  [unwired: 2 in, 2 out]
    n156 = node-c288() -> ()  [unwired: 1 in, 1 out]
  }
  n157 = control-ref of="C"() -> (w10:refnum<vi>)
  n158 = call-by-ref "Start Asynchronous Call"(reference=w5, "Stop signaller"=w3, "Fit parameters refnum"=w9, "C refnum"=w10, "Physical constants refnum"=w11, "Simulation parameters semaphore"=w4) -> (reference out=w2:refnum<vi>)  [unwired: 12 in, 1 out]
  n159 = while {
    tunnel: w3 -> [w285]
    tunnel: w22 -> [w284]
    tunnel: w21 -> [w283]
    tunnel: w12 -> [w282]
    tunnel: w2 -> [w281]
    tunnel: w1 -> [w280]
    stop <- w287 stop-if-true
    # "Check to see if we need to do something\nwith a configuration file"
    n160 = call "Peek or default.vi"("Signaller in"=w285) -> ("Has signal?"=w287:bool)  [unwired: 8 in, 2 out]
    n161 = Get Queue Status(queue=w280) -> (queue out=w278:refnum<queue>, # elements in queue=w277:i32)  [unwired: 2 in, 6 out]
    n162 = event shown="[1] \"Launch fit parameters chooser\": Value Change" {
      selector: _ -> [_ _ _ _ _ _ _ _ _ _]
      dyn-events: _ -> [_ _ _ _ _ _ _ _ _ _]
      timeout: 50 -> [_ _ _ _ _ _ _ _ _ _]
      tunnel: w285 -> [_ _ _ _ _ _ _ _ _ w404]
      tunnel: w284 -> [_ _ _ w395 _ _ _ _ _ _]
      tunnel: w283 -> [_ _ _ _ _ _ _ _ _ w403]
      tunnel: w282 -> [_ _ _ _ _ _ _ _ w402 _]
      tunnel: w281 -> [_ w390 _ _ _ _ _ _ _ _]
      event Timeout {
        n163 = event-data() -> ()  [unwired: 1 in, 3 out]
      }
      event "Launch fit parameters chooser": Value Change {
        # "Launch the fit parameters chooser\nif it has not already been launched"
        n164 = event-data() -> ()  [unwired: 1 in, 6 out]
        n165 = invoke class="VI Interface Type 0" method="FP.Open"(reference=w390) -> ()  [unwired: 4 in, 5 out]
      }
      event "Data output file": Value Change {
        # "Copy this value to the motor controller\ndata input file path for convenience\n(shouldn't have to set the same path\ntwice)"
        n166 = event-data() -> ()  [unwired: 1 in, 6 out]
        n167 = Not A Number/Path/Refnum?(number/path/refnum="Data input file refnum") -> (NaN/Path/Refnum?=w392:bool)
        n168 = case shown="False" w392 {
          tunnel: "Data input file refnum" -> [w394 _]
          frame False {
            n169 = property on="Data output file" class="Path"() -> ("Value"=w393:path)  [unwired: 2 in, 2 out]
            n170 = property class="Path"(reference=w394, "Value"=w393) -> ()  [unwired: 1 in, 2 out]
          }
          frame True {
          }
        }
      }
      event "Time scale (min)": Value Change {
        n171 = event-data() -> ()  [unwired: 1 in, 6 out]
        n172 = call "Signal.vi"("Signaller in"=w395) -> ()  [unwired: 9 in, 2 out]
      }
      event "5 minutes": Value Change {
        n173 = event-data() -> ()  [unwired: 1 in, 6 out]
        n174 = property on="Time scale (min)" class="DigNum (strict)"("Val(Sgnl)"=i64 5 ("Value (Signaling)")) -> ()  [unwired: 2 in, 2 out]
      }
      event "15 minutes": Value Change {
        n175 = event-data() -> ()  [unwired: 1 in, 6 out]
        n176 = property on="Time scale (min)" class="DigNum (strict)"("Val(Sgnl)"=i64 15 ("Value (Signaling)")) -> ()  [unwired: 2 in, 2 out]
      }
      event "30 minutes": Value Change {
        n177 = event-data() -> ()  [unwired: 1 in, 6 out]
        n178 = property on="Time scale (min)" class="DigNum (strict)"("Val(Sgnl)"=i64 30 ("Value (Signaling)")) -> ()  [unwired: 2 in, 2 out]
      }
      event "Add 30 minutes": Value Change {
        n179 = event-data() -> ()  [unwired: 1 in, 6 out]
        n180 = property on="Time scale (min)" class="DigNum (strict)"() -> ("Value"=w401:i64)  [unwired: 2 in, 2 out]
        n181 = Add(x=w401, y=i64 30) -> (x+y=w399:i64)
        n182 = property on="Time scale (min)" class="DigNum (strict)"("Val(Sgnl)"=w399) -> ()  [unwired: 2 in, 2 out]
      }
      event "Reset simulation": Value Change {
        n183 = event-data() -> ()  [unwired: 1 in, 6 out]
        n184 = call "Signal.vi"("Signaller in"=w402) -> ()  [unwired: 9 in, 2 out]
      }
      event "Stop simulation": Value Change {
        n185 = event-data() -> ()  [unwired: 1 in, 6 out]
        n186 = case shown="False" w403 {
          tunnel: w404 -> [w405 _]
          frame False {
            n187 = call "Signal.vi"("Signaller in"=w405) -> ()  [unwired: 9 in, 2 out]
          }
          frame True {
          }
        }
      }
    }
    n188 = Not Equal To 0?(x=w277) -> (x != 0?=w279:bool)
    n189 = case shown="True" w279 {
      tunnel: w278 -> [_ w291]
      frame False {
      }
      frame True {
        n190 = Dequeue Element(queue=w291) -> (element=w290:cluster{path, bool})  [unwired: 2 in, 3 out]
        n191 = Unbundle(w290) -> (w288:path, w289:bool)
        n192 = case shown="False" w289 {
          tunnel: w288 -> [w346 w389]
          frame False {
            w331 = "Simulation" ("section")
            # "Restore configuration from file"
            n193 = property on="Data output file" class="Path"() -> ("Value"=w330:path)  [unwired: 2 in, 2 out]
            n194 = call <vilib>:"Open Config Data.vi"("create file if necessary (T)"=FALSE, "configuration file path"=w346) -> ("refnum"=w345:T11)  [unwired: 7 in, 2 out]
            n195 = call-poly <vilib>:"Read Key.vi"("section"=w331, "default value"=w330, "key"="Data output file", "refnum"=w345) -> ("value"=w329:path, "refnum out"=w344:T11)  [unwired: 4 in, 2 out]
            n196 = property on="Data output file" class="Path"("Value"=w329) -> ()  [unwired: 2 in, 2 out]
            n197 = property on="Beam on" class="Bool (strict)"() -> ("Value"=w327:bool)  [unwired: 2 in, 2 out]
            n198 = call-poly <vilib>:"Read Key.vi"("section"=w331, "default value"=w327, "key"="Beam on", "refnum"=w344) -> ("value"=w325:bool, "refnum out"=w343:T11)  [unwired: 4 in, 2 out]
            n199 = property on="Beam on" class="Bool (strict)"("Value"=w325) -> ()  [unwired: 2 in, 2 out]
            n200 = property on="A" class="DigNum (strict)"() -> ("Value"=w324:dbl)  [unwired: 2 in, 2 out]
            n201 = call-poly <vilib>:"Read Key.vi"("section"=w331, "default value"=w324, "key"="A", "refnum"=w343) -> ("value"=w322:dbl, "refnum out"=w342:T11)  [unwired: 4 in, 2 out]
            n202 = property on="A" class="DigNum (strict)"("Value"=w322) -> ()  [unwired: 2 in, 2 out]
            n203 = property on="S" class="DigNum (strict)"() -> ("Value"=w320:dbl)  [unwired: 2 in, 2 out]
            n204 = call-poly <vilib>:"Read Key.vi"("section"=w331, "default value"=w320, "key"="S", "refnum"=w342) -> ("value"=w319:dbl, "refnum out"=w341:T11)  [unwired: 4 in, 2 out]
            n205 = property on="S" class="DigNum (strict)"("Value"=w319) -> ()  [unwired: 2 in, 2 out]
            n206 = property on="M1" class="DigNum (strict)"() -> ("Value"=w316:dbl)  [unwired: 2 in, 2 out]
            n207 = call-poly <vilib>:"Read Key.vi"("section"=w331, "default value"=w316, "key"="M1", "refnum"=w341) -> ("value"=w318:dbl, "refnum out"=w340:T11)  [unwired: 4 in, 2 out]
            n208 = property on="M1" class="DigNum (strict)"("Value"=w318) -> ()  [unwired: 2 in, 2 out]
            n209 = property on="M2" class="DigNum (strict)"() -> ("Value"=w313:dbl)  [unwired: 2 in, 2 out]
            n210 = call-poly <vilib>:"Read Key.vi"("section"=w331, "default value"=w313, "key"="M2", "refnum"=w340) -> ("value"=w314:dbl, "refnum out"=w339:T11)  [unwired: 4 in, 2 out]
            n211 = property on="M2" class="DigNum (strict)"("Value"=w314) -> ()  [unwired: 2 in, 2 out]
            n212 = property on="C" class="DigNum (strict)"() -> ("Value"=w311:dbl)  [unwired: 2 in, 2 out]
            n213 = call-poly <vilib>:"Read Key.vi"("section"=w331, "default value"=w311, "key"="C", "refnum"=w339) -> ("value"=w310:dbl, "refnum out"=w338:T11)  [unwired: 4 in, 2 out]
            n214 = property on="C" class="DigNum (strict)"("Value"=w310) -> ()  [unwired: 2 in, 2 out]
            n215 = property on="T1e (s)" class="DigNum (strict)"() -> ("Value"=w308:dbl)  [unwired: 2 in, 2 out]
            n216 = call-poly <vilib>:"Read Key.vi"("section"=w331, "default value"=w308, "key"="T1e", "refnum"=w338) -> ("value"=w307:dbl, "refnum out"=w337:T11)  [unwired: 4 in, 2 out]
            n217 = property on="T1e (s)" class="DigNum (strict)"("Value"=w307) -> ()  [unwired: 2 in, 2 out]
            n218 = property on="T1n (s)" class="DigNum (strict)"() -> ("Value"=w306:dbl)  [unwired: 2 in, 2 out]
            n219 = call-poly <vilib>:"Read Key.vi"("section"=w331, "default value"=w306, "key"="T1n", "refnum"=w337) -> ("value"=w304:dbl, "refnum out"=w336:T11)  [unwired: 4 in, 2 out]
            n220 = property on="T1n (s)" class="DigNum (strict)"("Value"=w304) -> ()  [unwired: 2 in, 2 out]
            n221 = property on="# Sweeps" class="DigNum (strict)"() -> ("Value"=w302:u32)  [unwired: 2 in, 2 out]
            n222 = property on="Thermal fluctuations" class="DigNum (strict)"() -> ("Value"=w300:dbl)  [unwired: 2 in, 2 out]
            n223 = call-poly <vilib>:"Read Key.vi"("section"=w331, "default value"=w302, "key"="Number of sweeps", "refnum"=w336) -> ("value"=w301:u32, "refnum out"=w335:T11)  [unwired: 4 in, 2 out]
            n224 = property on="# Sweeps" class="DigNum (strict)"("Value"=w301) -> ()  [unwired: 2 in, 2 out]
            n225 = property on="Sweep error" class="DigNum (strict)"() -> ("Value"=w296:dbl)  [unwired: 2 in, 2 out]
            n226 = call-poly <vilib>:"Read Key.vi"("section"=w331, "default value"=w300, "key"="Thermal fluctuations", "refnum"=w335) -> ("value"=w298:dbl, "refnum out"=w334:T11)  [unwired: 4 in, 2 out]
            n227 = property on="Thermal fluctuations" class="DigNum (strict)"("Value"=w298) -> ()  [unwired: 2 in, 2 out]
            n228 = call-poly <vilib>:"Read Key.vi"("section"=w331, "default value"=w296, "key"="Sweep error", "refnum"=w334) -> ("value"=w295:dbl, "refnum out"=w333:T11)  [unwired: 4 in, 2 out]
            n229 = property on="Sweep error" class="DigNum (strict)"("Value"=w295) -> ()  [unwired: 2 in, 2 out]
            n230 = property on="Precision" class="DigNum (strict)"() -> ("Value"=w294:i32)  [unwired: 2 in, 2 out]
            n231 = call-poly <vilib>:"Read Key.vi"("section"=w331, "default value"=w294, "key"="Precision", "refnum"=w333) -> ("value"=w292:i32, "refnum out"=w332:T11)  [unwired: 4 in, 2 out]
            n232 = property on="Precision" class="DigNum (strict)"("Value"=w292) -> ()  [unwired: 2 in, 2 out]
            n233 = call <vilib>:"Close Config Data.vi"("refnum"=w332) -> ()  [unwired: 9 in, 2 out]
          }
          frame True {
            w375 = "Simulation" ("section")
            # "Save configuration to file"
            n234 = property on="Data output file" class="Path"() -> ("Value"=w373:path)  [unwired: 2 in, 2 out]
            n235 = call <vilib>:"Open Config Data.vi"("configuration file path"=w389) -> ("refnum"=w388:T11)  [unwired: 8 in, 2 out]
            n236 = call-poly <vilib>:"Write Key.vi"("section"=w375, "value"=w373, "key"="Data output file", "refnum"=w388) -> ("refnum out"=w387:T11)  [unwired: 5 in, 2 out]
            n237 = property on="Beam on" class="Bool (strict)"() -> ("Value"=w371:bool)  [unwired: 2 in, 2 out]
            n238 = call-poly <vilib>:"Write Key.vi"("section"=w375, "value"=w371, "key"="Beam on", "refnum"=w387) -> ("refnum out"=w386:T11)  [unwired: 5 in, 2 out]
            n239 = property on="A" class="DigNum (strict)"() -> ("Value"=w348:dbl)  [unwired: 2 in, 2 out]
            n240 = call-poly <vilib>:"Write Key.vi"("section"=w375, "value"=w348, "key"="A", "refnum"=w386) -> ("refnum out"=w385:T11)  [unwired: 5 in, 2 out]
            n241 = property on="S" class="DigNum (strict)"() -> ("Value"=w368:dbl)  [unwired: 2 in, 2 out]
            n242 = call-poly <vilib>:"Write Key.vi"("section"=w375, "value"=w368, "key"="S", "refnum"=w385) -> ("refnum out"=w384:T11)  [unwired: 5 in, 2 out]
            n243 = property on="M1" class="DigNum (strict)"() -> ("Value"=w366:dbl)  [unwired: 2 in, 2 out]
            n244 = call-poly <vilib>:"Write Key.vi"("section"=w375, "value"=w366, "key"="M1", "refnum"=w384) -> ("refnum out"=w383:T11)  [unwired: 5 in, 2 out]
            n245 = property on="M2" class="DigNum (strict)"() -> ("Value"=w364:dbl)  [unwired: 2 in, 2 out]
            n246 = call-poly <vilib>:"Write Key.vi"("section"=w375, "value"=w364, "key"="M2", "refnum"=w383) -> ("refnum out"=w382:T11)  [unwired: 5 in, 2 out]
            n247 = property on="C" class="DigNum (strict)"() -> ("Value"=w362:dbl)  [unwired: 2 in, 2 out]
            n248 = call-poly <vilib>:"Write Key.vi"("section"=w375, "value"=w362, "key"="C", "refnum"=w382) -> ("refnum out"=w381:T11)  [unwired: 5 in, 2 out]
            n249 = property on="T1e (s)" class="DigNum (strict)"() -> ("Value"=w360:dbl)  [unwired: 2 in, 2 out]
            n250 = call-poly <vilib>:"Write Key.vi"("section"=w375, "value"=w360, "key"="T1e", "refnum"=w381) -> ("refnum out"=w380:T11)  [unwired: 5 in, 2 out]
            n251 = property on="T1n (s)" class="DigNum (strict)"() -> ("Value"=w358:dbl)  [unwired: 2 in, 2 out]
            n252 = call-poly <vilib>:"Write Key.vi"("section"=w375, "value"=w358, "key"="T1n", "refnum"=w380) -> ("refnum out"=w379:T11)  [unwired: 5 in, 2 out]
            n253 = property on="# Sweeps" class="DigNum (strict)"() -> ("Value"=w356:u32)  [unwired: 2 in, 2 out]
            n254 = property on="Thermal fluctuations" class="DigNum (strict)"() -> ("Value"=w354:dbl)  [unwired: 2 in, 2 out]
            n255 = call-poly <vilib>:"Write Key.vi"("section"=w375, "value"=w356, "key"="Number of sweeps", "refnum"=w379) -> ("refnum out"=w378:T11)  [unwired: 5 in, 2 out]
            n256 = property on="Sweep error" class="DigNum (strict)"() -> ("Value"=w352:dbl)  [unwired: 2 in, 2 out]
            n257 = call-poly <vilib>:"Write Key.vi"("section"=w375, "value"=w354, "key"="Thermal fluctuations", "refnum"=w378) -> ("refnum out"=w377:T11)  [unwired: 5 in, 2 out]
            n258 = call-poly <vilib>:"Write Key.vi"("section"=w375, "value"=w352, "key"="Sweep error", "refnum"=w377) -> ("refnum out"=w376:T11)  [unwired: 5 in, 2 out]
            n259 = property on="Precision" class="DigNum (strict)"() -> ("Value"=w350:i32)  [unwired: 2 in, 2 out]
            n260 = call-poly <vilib>:"Write Key.vi"("section"=w375, "value"=w350, "key"="Precision", "refnum"=w376) -> ("refnum out"=w349:T11)  [unwired: 5 in, 2 out]
            n261 = call <vilib>:"Close Config Data.vi"("refnum"=w349) -> ()  [unwired: 9 in, 2 out]
          }
        }
      }
    }
  }
  n262 = node-c288(w35) -> ()  [unwired: 1 out]
  n263 = node-c288(w33) -> ()  [unwired: 1 out]
  n264 = node-c288(w26) -> ()  [unwired: 1 out]
  n265 = node-c288(w37) -> ()  [unwired: 1 out]
  n266 = call "Destroy.vi"("Signaller in"=w13) -> ()  [unwired: 10 in, 1 out]
  n267 = call "Destroy.vi"("Signaller in"=w29) -> ()  [unwired: 10 in, 1 out]
  n268 = call "Destroy.vi"("Signaller in"=w25) -> ()  [unwired: 10 in, 1 out]
